vi "Obtain_arrays.vi"(10 "Q Graph":cluster{"Array":dbl[], "Array 2":dbl[]}, 11 "P Graph and Intensities and RF":cluster{"Array":dbl[], "Array":dbl[]}[](array[cluster])) -> (0 "RF Range 2":dbl[](array[numeric]), 1 "RF Range 1":dbl[](array[numeric]), 2 "Q":dbl[](array[numeric]), 3 "P":dbl[](array[numeric]), 4 "I+":dbl[](array[numeric]), 6 "I-":dbl[](array[numeric]), 8 "AFP Range":dbl[](array[numeric]))   [LabVIEW 2018]
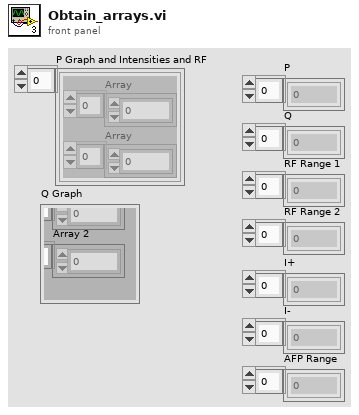
[diagram p1: front panel]
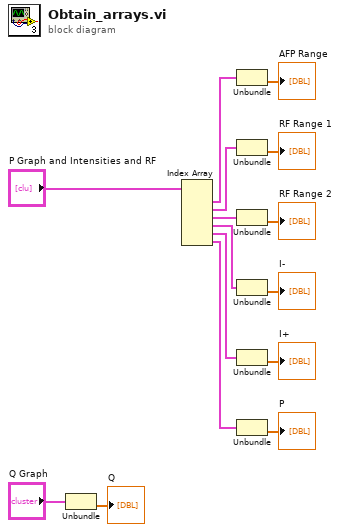
[diagram p0: block diagram]
diagram:
  n1 = Unbundle("Q Graph") -> ("Array 2"=→"Q":dbl[])  [unwired: 1 out]
  n2 = Index Array(array="P Graph and Intensities and RF") -> (element #1=w13:cluster{"Array":dbl[], "Array":dbl[]}, element #2=w12:cluster{"Array":dbl[], "Array":dbl[]}, element #3=w8:cluster{"Array":dbl[], "Array":dbl[]}, element #4=w9:cluster{"Array":dbl[], "Array":dbl[]}, element #5=w10:cluster{"Array":dbl[], "Array":dbl[]}, element #6=w11:cluster{"Array":dbl[], "Array":dbl[]})  [unwired: 6 in]
  n3 = Unbundle(w13) -> ("Array"=→"AFP Range":dbl[])  [unwired: 1 out]
  n4 = Unbundle(w12) -> ("Array"=→"RF Range 1":dbl[])  [unwired: 1 out]
  n5 = Unbundle(w8) -> ("Array"=→"RF Range 2":dbl[])  [unwired: 1 out]
  n6 = Unbundle(w9) -> ("Array"=→"I-":dbl[])  [unwired: 1 out]
  n7 = Unbundle(w10) -> ("Array"=→"I+":dbl[])  [unwired: 1 out]
  n8 = Unbundle(w11) -> ("Array"=→"P":dbl[])  [unwired: 1 out]
